vi "Specify Delete Action.vi"(11 "Subscription in":refnum<class "Subscription.lvclass">) -> (2 "Delete action":string, 3 "Subscription out":refnum<class "Subscription.lvclass">)   [LabVIEW 2015, in "NI_AWS_SNS.lvlib" / "Subscription.lvclass"]
uses:
  Subscription.lvclass
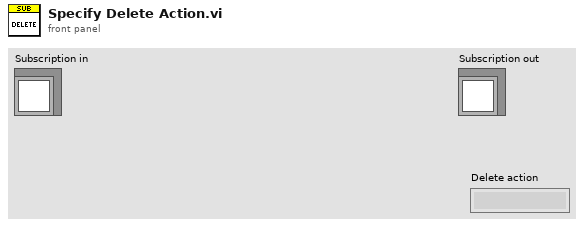
[diagram p1: front panel]
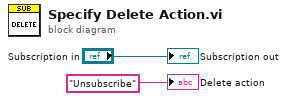
[diagram p0: block diagram]
diagram:
  "Subscription out" <- "Subscription in"
  "Delete action" <- "Unsubscribe" ("value")
